vi "Save Digital Patterns - Multi FPGA.vi"(8 "error in (no error)":errorcluster, 10 "Patterns":T1[](array[typedef]), 11 "Item Ref in":T5 format="%.0x") -> (0 "error out":errorcluster)   [LabVIEW 2015, in "Engine Simulation Toolkit System Explorer.lvlib"]
uses:
  Engine Simulation Toolkit System Explorer.lvlib
  <vilib>/NI Veristand/Custom Device API/Custom Device Item Ref.ctl
  Digital Pattern.ctl
  Digital Pattern Base.ctl
  Digital Pattern Remove Edge.ctl
  Digital Pattern Add Pulse.ctl
  Shared/Properties.vi
  <vilib>/NI Veristand/Custom Device API/Set Item Property (String).vi
  <vilib>/NI Veristand/Custom Device API/Set Item Property (Double).vi
  <vilib>/NI Veristand/Custom Device API/Set Item Property (U16).vi
  <vilib>/NI Veristand/Custom Device API/Set Item Property (Boolean).vi
  Shared/Engine Simulation Toolkit Shared.lvlib
  <vilib>/NI Veristand/Custom Device API/Custom Device API.lvlib
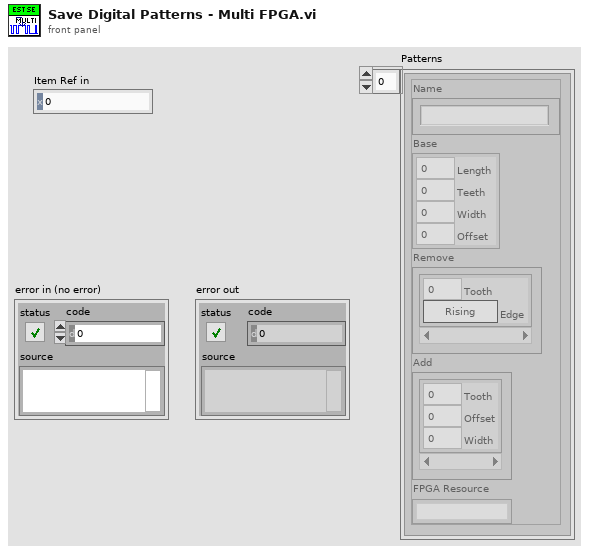
[diagram p1: front panel]
types:
  T1 = typedef "Engine Simulation Toolkit System Explorer.lvlib/Digital Pattern.ctl" = cluster{"Name":string, "Base":T2, "Remove":T3[], "Add":T4[], "FPGA Resource":string}
  T2 = typedef "Engine Simulation Toolkit System Explorer.lvlib/Digital Pattern Base.ctl" = cluster{"Length":dbl, "Teeth":u16, "Width":dbl, "Offset":dbl}
  T3 = typedef "Engine Simulation Toolkit System Explorer.lvlib/Digital Pattern Remove Edge.ctl" = cluster{"Tooth":u16, "Edge":bool}
  T4 = typedef "Engine Simulation Toolkit System Explorer.lvlib/Digital Pattern Add Pulse.ctl" = cluster{"Tooth":u16, "Offset":dbl, "Width":dbl}
  T5 = typedef "Custom Device API.lvlib/Custom Device Item Ref.ctl" = u64
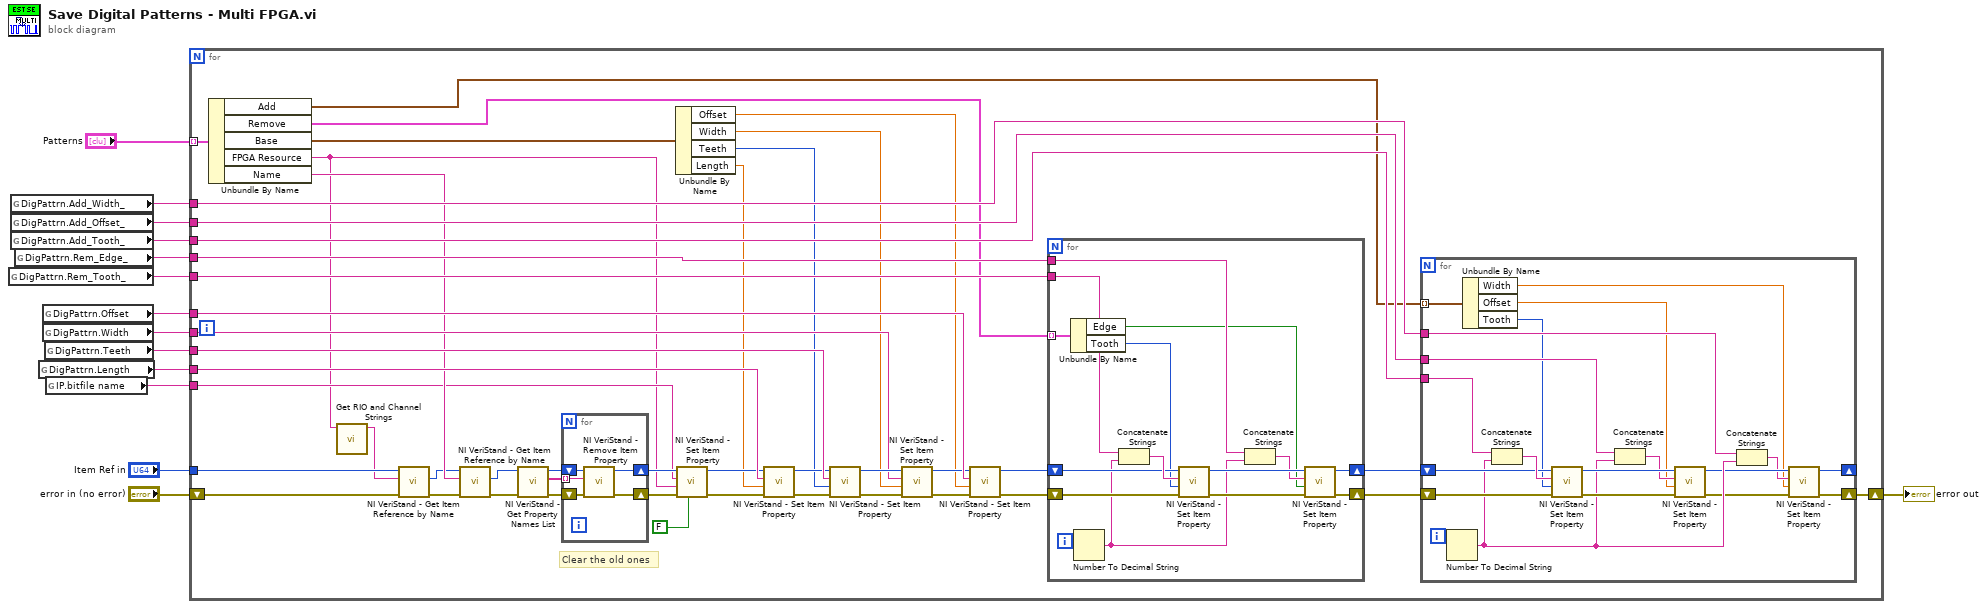
[diagram p0: block diagram]
diagram:
  n1 = global read "Properties.vi" "DigPattrn.Rem_Tooth_"() -> (w8:string)
  n2 = global read "Properties.vi" "DigPattrn.Add_Width_"() -> (w6:string)
  n3 = global read "Properties.vi" "DigPattrn.Add_Offset_"() -> (w5:string)
  n4 = global read "Properties.vi" "DigPattrn.Add_Tooth_"() -> (w4:string)
  n5 = global read "Properties.vi" "DigPattrn.Rem_Edge_"() -> (w7:string)
  n6 = global read "Properties.vi" "DigPattrn.Length"() -> (w12:string)
  n7 = global read "Properties.vi" "DigPattrn.Offset"() -> (w9:string)
  n8 = global read "Properties.vi" "DigPattrn.Width"() -> (w10:string)
  n9 = global read "Properties.vi" "DigPattrn.Teeth"() -> (w11:string)
  n10 = global read "Properties.vi" "IP.bitfile name"() -> (w1:string)
  n11 = for {
    shift-right: [w53] -> w13
    shift-left: "error in (no error)" -> [w19]
    tunnel: w12 -> [w60]
    tunnel: w11 -> [w59]
    tunnel: w10 -> [w42]
    tunnel: w9 -> [w58]
    tunnel: w8 -> [w57]
    tunnel: w7 -> [w56]
    tunnel: w4 -> [w54]
    tunnel: w5 -> [w41]
    tunnel: w6 -> [w55]
    tunnel: "Item Ref in" -> [w17]
    tunnel: "Patterns" -> [w40] mode=indexing
    tunnel: w1 -> [w28]
    # "Clear the old ones"
    n12 = Unbundle By Name(w40) -> ("Add"=w22:T4[], "Remove"=w23:T3[], "Base"=w37:T2, "FPGA Resource"=w16:string, "Name"=w38:string)
    n13 = call "Get RIO and Channel Strings.vi"("rio/analog replay"=w16) -> ("rio"=w15:string)  [unwired: 9 in, 1 out]
    n14 = call <vilib>:"NI VeriStand - Get Item Reference by Name.vi"("error in (no error)"=w19, "Item Name"=w15, "Parent Ref in"=w17) -> ("error out"=w20:errorcluster, "Item Ref"=w18:T5)  [unwired: 5 in, 2 out]
    n15 = call <vilib>:"NI VeriStand - Get Item Reference by Name.vi"("error in (no error)"=w20, "Item Name"=w38, "Parent Ref in"=w18) -> ("error out"=w39:errorcluster, "Item Ref"=w35:T5)  [unwired: 5 in, 2 out]
    n16 = call <vilib>:"NI VeriStand - Get Property Names List.vi"("error in (no error)"=w39, "Item Ref in"=w35) -> ("error out"=w36:errorcluster, "Property Names"=w32:string[], "Item Ref out"=w33:T5)  [unwired: 7 in]
    n17 = for {
      tunnel: w32 -> [w96] mode=indexing
      shift-right: [w97] -> w30
      shift-left: w33 -> [w98]
      shift-right: [w99] -> w34
      shift-left: w36 -> [w100]
      n18 = call <vilib>:"NI VeriStand - Remove Item Property.vi"("error in (no error)"=w100, "Property Name"=w96, "Item Ref in"=w98) -> ("error out"=w99:errorcluster, "Item Ref out"=w97:T5)  [unwired: 6 in, 1 out]
    }
    n19 = Unbundle By Name(w37) -> ("Offset"=w24:dbl, "Width"=w25:dbl, "Teeth"=w26:u16, "Length"=w27:dbl)
    n20 = call-poly <vilib>:"NI VeriStand - Set Item Property.vi"("Binary String (T)"=FALSE, "error in (no error)"=w34, "Value"=w16, "Property Name"=w28, "Item Ref in"=w30) -> ("error out"=w31:errorcluster, "Item Ref out"=w29:T5)  [unwired: 4 in, 1 out]
    n21 = call-poly <vilib>:"NI VeriStand - Set Item Property.vi"("error in (no error)"=w31, "Value"=w27, "Property Name"=w60, "Item Ref in"=w29) -> ("error out"=w51:errorcluster, "Item Ref out"=w52:T5)  [unwired: 5 in, 1 out]
    n22 = call-poly <vilib>:"NI VeriStand - Set Item Property.vi"("error in (no error)"=w51, "Value"=w26, "Property Name"=w59, "Item Ref in"=w52) -> ("error out"=w49:errorcluster, "Item Ref out"=w50:T5)  [unwired: 5 in, 1 out]
    n23 = call-poly <vilib>:"NI VeriStand - Set Item Property.vi"("error in (no error)"=w49, "Value"=w25, "Property Name"=w42, "Item Ref in"=w50) -> ("error out"=w47:errorcluster, "Item Ref out"=w48:T5)  [unwired: 5 in, 1 out]
    n24 = call-poly <vilib>:"NI VeriStand - Set Item Property.vi"("error in (no error)"=w47, "Value"=w24, "Property Name"=w58, "Item Ref in"=w48) -> ("error out"=w43:errorcluster, "Item Ref out"=w44:T5)  [unwired: 5 in, 1 out]
    n25 = for {
      shift-right: [w85] -> w45
      shift-left: w43 -> [w93]
      shift-right: [w86] -> w46
      shift-left: w44 -> [w94]
      tunnel: w56 -> [w89]
      tunnel: w57 -> [w87]
      tunnel: w23 -> [w83] mode=indexing
      i -> [w92]
      n26 = Unbundle By Name(w83) -> ("Edge"=w81:bool, "Tooth"=w82:u16)
      n27 = Number To Decimal String(number=w92) -> (decimal integer string=w88:string)  [unwired: 1 in]
      n28 = Concatenate Strings(w87, w88) -> (w95:string)
      n29 = call-poly <vilib>:"NI VeriStand - Set Item Property.vi"("error in (no error)"=w93, "Value"=w82, "Property Name"=w95, "Item Ref in"=w94) -> ("error out"=w91:errorcluster, "Item Ref out"=w90:T5)  [unwired: 5 in, 1 out]
      n30 = Concatenate Strings(w89, w88) -> (w84:string)
      n31 = call-poly <vilib>:"NI VeriStand - Set Item Property.vi"("error in (no error)"=w91, "Value"=w81, "Property Name"=w84, "Item Ref in"=w90) -> ("error out"=w85:errorcluster, "Item Ref out"=w86:T5)  [unwired: 5 in, 1 out]
    }
    n32 = for {
      shift-right: [w70] -> w53
      shift-left: w45 -> [w78]
      shift-right: [w71] -> _
      shift-left: w46 -> [w79]
      tunnel: w41 -> [w74]
      tunnel: w54 -> [w72]
      tunnel: w55 -> [w69]
      tunnel: w22 -> [w64] mode=indexing
      i -> [w77]
      n33 = Number To Decimal String(number=w77) -> (decimal integer string=w73:string)  [unwired: 1 in]
      n34 = Unbundle By Name(w64) -> ("Width"=w61:dbl, "Offset"=w62:dbl, "Tooth"=w63:u16)
      n35 = Concatenate Strings(w72, w73) -> (w80:string)
      n36 = call-poly <vilib>:"NI VeriStand - Set Item Property.vi"("error in (no error)"=w78, "Value"=w63, "Property Name"=w80, "Item Ref in"=w79) -> ("error out"=w76:errorcluster, "Item Ref out"=w75:T5)  [unwired: 5 in, 1 out]
      n37 = Concatenate Strings(w74, w73) -> (w68:string)
      n38 = call-poly <vilib>:"NI VeriStand - Set Item Property.vi"("error in (no error)"=w76, "Value"=w62, "Property Name"=w68, "Item Ref in"=w75) -> ("error out"=w66:errorcluster, "Item Ref out"=w67:T5)  [unwired: 5 in, 1 out]
      n39 = Concatenate Strings(w69, w73) -> (w65:string)
      n40 = call-poly <vilib>:"NI VeriStand - Set Item Property.vi"("error in (no error)"=w66, "Value"=w61, "Property Name"=w65, "Item Ref in"=w67) -> ("error out"=w70:errorcluster, "Item Ref out"=w71:T5)  [unwired: 5 in, 1 out]
    }
  }
  "error out" <- w13
